vi "Numeric Case Structures.vi"() -> ()   [LabVIEW 2019]
panel:
  in  "Mode":i32
  in  "stop":bool
  out "Temperature Output":dbl(slide) scale=0.0..212.0
  in  "Celsius Input":dbl(slide) scale=-200.0..100.0
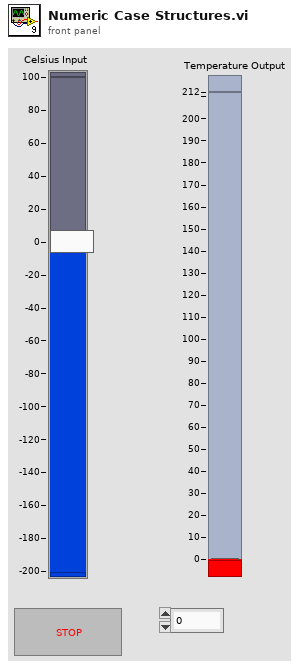
[diagram p1: front panel]
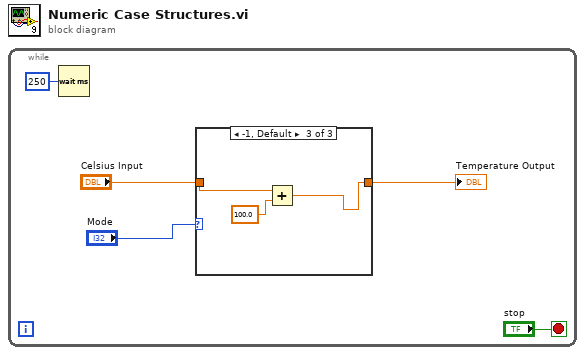
[diagram p0: block diagram]
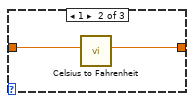
[diagram p3: hidden frame]
diagram:
  n1 = while {
    stop <- "stop" stop-if-true
    n2 = Wait (ms)(milliseconds to wait=u32 250) -> ()  [unwired: 1 out]
    n3 = case shown="-1, Default" "Mode" {
      tunnel: "Celsius Input" -> [w6 w8 w9]
      tunnel: [w6 w7 w10] -> w4
      frame 0 {
      }
      frame 1 {
        n4 = call "Celsius to Fahrenheit.vi"("Celsius"=w8) -> ("Fahrenheit"=w7:dbl)  [unwired: 10 in]
      }
      frame -1, Default {
        n5 = Add(x=w9, y=100.0) -> (x+y=w10:dbl)
      }
    }
    "Temperature Output" <- w4
  }
